vi "Complete Request.vi"(7 "Processing In":refnum<class "Processing.lvclass">, 11 "Complete Handler in":refnum<class "Complete Handler.lvclass">) -> (0 "error out":errorcluster, 5 "Processing":refnum<class "Processing.lvclass">)   [LabVIEW 2020, in "HTTP Server.lvlib" / "Complete Handler.lvclass"]
uses:
  Complete Handler.lvclass
  Processing/Processing.lvclass
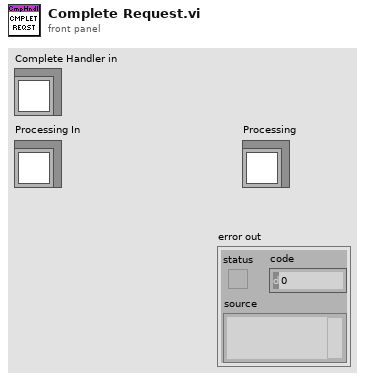
[diagram p1: front panel]
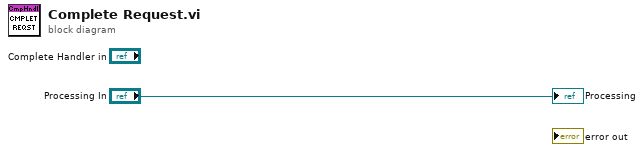
[diagram p0: block diagram]
diagram:
  "Processing" <- "Processing In"
